vi "resonance monitor control.vi"() -> ()   [LabVIEW 2014]
uses:
  resonance monitor ctl action.ctl
  interpolation state - real.ctl
  peak monitor ctl - V2.ctl
panel:
  out "All Objects[]":refnum<vi>[](array[refnum])
  out "peak monitor ctl ref OUT":refnum<vi>
  in  "peak monitor ctl ref IN":refnum<vi>
  in  "resonance monitor ctl action":T1
  in  "peak monitor ctl":T2={"delta"=0.0, "gamma"=0.0, "exp"=0.0, "found?"=FALSE, "found"=0.0, "gamma found"=0.0, "init linear"=FALSE, "interpolate"=enum."last", "gamma-factor"=3.5, "slope"=0.0, "update freq?"=FALSE, "update gamma?"=FALSE, "acc factor"=3.5, "linear interpolation state"={"requested size"=20, "Array"=[], "actual number of elements"=0}, "ind"=0.0, "gamma ratio"=0.0}
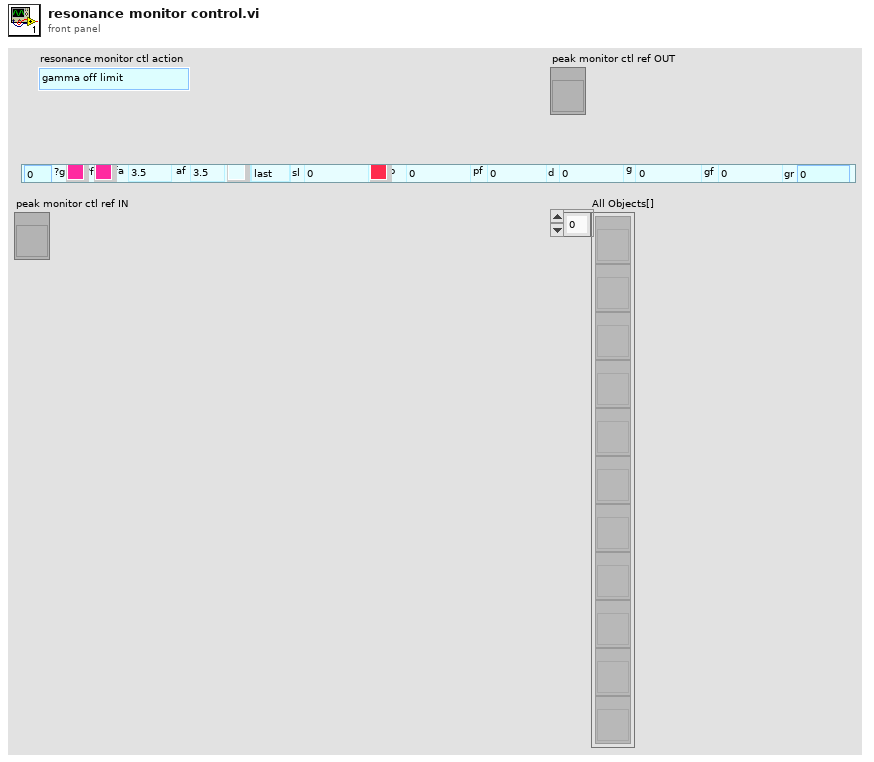
[diagram p1: front panel]
types:
  T1 = typedef "resonance monitor ctl action.ctl" = enum16{"gamma off limit", "void"}
  T2 = typedef "peak monitor ctl - V2.ctl" = cluster{"delta":dbl, "gamma":dbl, "exp":dbl, "found?":bool, "found":dbl, "gamma found":dbl, "init linear":bool, "interpolate":enum16{"line", "last"}, "gamma-factor":dbl, "slope":dbl, "update freq?":bool, "update gamma?":bool, "acc factor":dbl, "linear interpolation state":T3, "ind":dbl, "gamma ratio":dbl}
  T3 = typedef "interpolation state - real.ctl" = cluster{"requested size":i32, "Array":dbl[], "actual number of elements":i32}
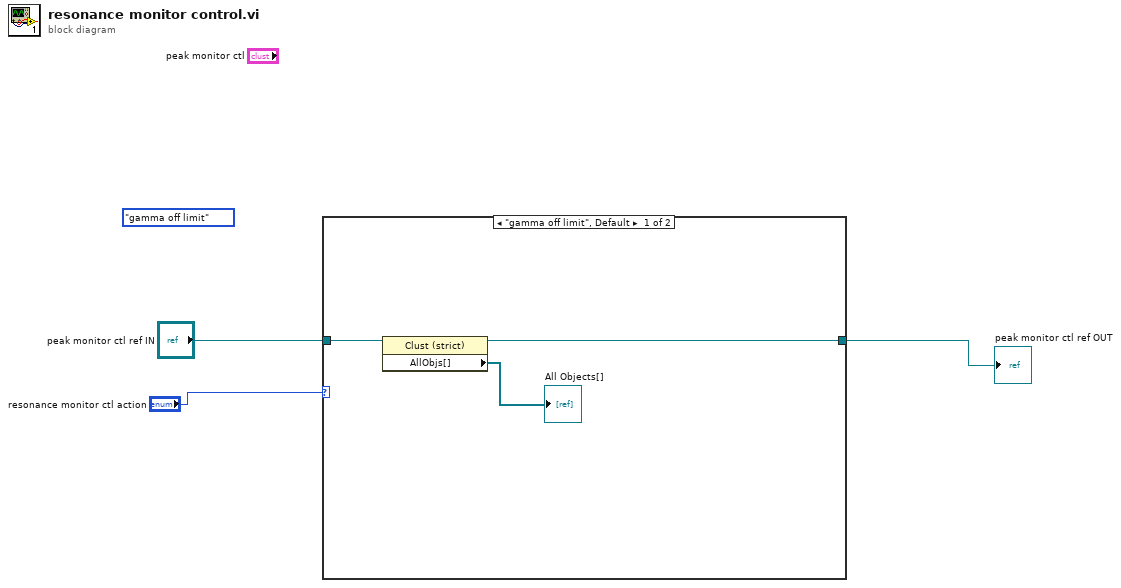
[diagram p0: block diagram]
diagram:
  (unwired) resonance_monitor_ctl_action."gamma off limit" ("resonance monitor ctl action")
  n1 = case shown="\"gamma off limit\", Default" "resonance monitor ctl action" {
    tunnel: "peak monitor ctl ref IN" -> [w6 _]
    tunnel: [w5 _] -> w1
    frame "gamma off limit", Default {
      n2 = property class="Clust (strict)"(reference=w6) -> (reference out=w5:refnum<vi>, "AllObjs[]"=→"All Objects[]":refnum<vi>[])  [unwired: 1 in, 1 out]
    }
    frame "void" {
    }
  }
  "peak monitor ctl ref OUT" <- w1
